vi "ifr2025 ILS  (not On Ifr2025).vi"(8 "error in (no error)":errorcluster {"code" format="%.0x"}, 11 "instrument handle":refnum<visa-resource-name>) -> (0 "error out":errorcluster {"code" format="%.0x"}, 1 "DDM Depth":dbl, 2 "SDM Depth":dbl, 3 "instrument handle out":refnum<visa-resource-name>, 4 "ILSID Depth":dbl, 5 "DDM Type":i16)   [LabVIEW 2009]
doc: "Retrieve the current settings for ILS mode."
uses:
  Ifr2025_32.dll
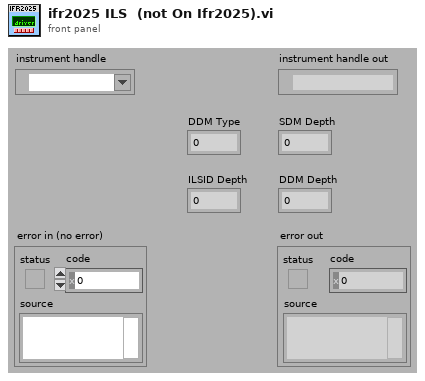
[diagram p1: front panel]
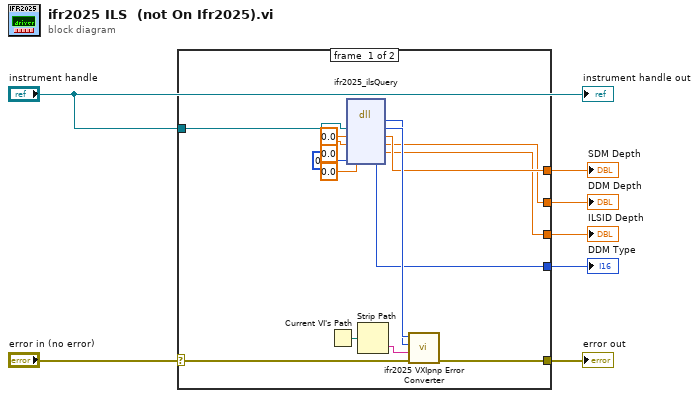
[diagram p0: block diagram]
diagram:
  n1 = case shown="No Error" "error in (no error)" {
    selector: "error in (no error)" -> [w17 w23]
    tunnel: [w16 w23] -> w7
    tunnel: "instrument handle" -> [w21 _]
    tunnel: [w14 _] -> w4
    tunnel: [w12 _] -> w3
    tunnel: [w10 _] -> w2
    tunnel: [w8 _] -> w1
    frame #0 {
      n2 = Current VI's Path() -> (path=w22:path)
      n3 = dll-call lib="P:/inst/Marconi 2024 Signal Generator/source/labview/ifr2025/ifr2025/ifr2025_*.*" fn="ifr2025_ilsQuery"("vi"=w21, "SDM Depth"=0.0, "DDM Depth"=0.0, "ILSID Depth"=0.0, "DDM Type"=i16 0) -> (w19:i32, "vi"=w20:u32, "SDM Depth"=w14:dbl, "DDM Depth"=w12:dbl, "ILSID Depth"=w10:dbl, "DDM Type"=w8:i16)  [unwired: 3 in, 2 out]
      n4 = Strip Path(path=w22) -> (name=w18:string)  [unwired: 1 out]
      n5 = call "ifr2025 VXIpnp Error Converter.vi"("error in (no error)"=w17, "name of VI (\"\")"=w18, "CVI error code (0)"=w19, "instrument handle"=w20) -> ("error out"=w16:errorcluster)  [unwired: 7 out]
    }
    frame #1 {
    }
  }
  "error out" <- w7
  "SDM Depth" <- w4
  "DDM Depth" <- w3
  "ILSID Depth" <- w2
  "DDM Type" <- w1
  "instrument handle out" <- "instrument handle"
